vi "Normalize Waveform.vi"(0 "Waveform In":T1={"Waveform Name"="Wfm", "Waveform"={"x0"=0.0, "dx"=0.0, "y"=[]}, "Signal Bandwidth (Hz)"=0.0, "PAPR (dB)"=0.0, "Burst Length (s)"=0.0, "Sample Rate"=0.0, "Burst Start Locations"=[], "Burst Stop Locations"=[], "Idle Duration Present?"=FALSE} {"Sample Rate" format="%#_6p"; "Burst Length (s)" format="%#_6p"; "PAPR (dB)" format="%.2f"; "Signal Bandwidth (Hz)" format="%.2f"; "Waveform"."y" format="%.2f"; "Waveform"."dx" format="%^.2e"; "Waveform"."x0" format="%^.2e"}) -> (4 "Waveform Out":T1={"Waveform Name"="Wfm", "Waveform"={"x0"=0.0, "dx"=0.0, "y"=[]}, "Signal Bandwidth (Hz)"=0.0, "PAPR (dB)"=0.0, "Burst Length (s)"=0.0, "Sample Rate"=0.0, "Burst Start Locations"=[], "Burst Stop Locations"=[], "Idle Duration Present?"=FALSE} {"Sample Rate" format="%#_6p"; "Burst Length (s)" format="%#_6p"; "PAPR (dB)" format="%.2f"; "Signal Bandwidth (Hz)" format="%.2f"; "Waveform"."y" format="%.2f"; "Waveform"."dx" format="%^.2e"; "Waveform"."x0" format="%^.2e"})   [LabVIEW 2018, in "SG.lvlib"]
uses:
  SG.lvlib
  Typedefs/Waveform.ctl
  <vilib>/Analysis/5stat.llb/RMS (CDB).vi
  <vilib>/Analysis/NI_AALPro.lvlib
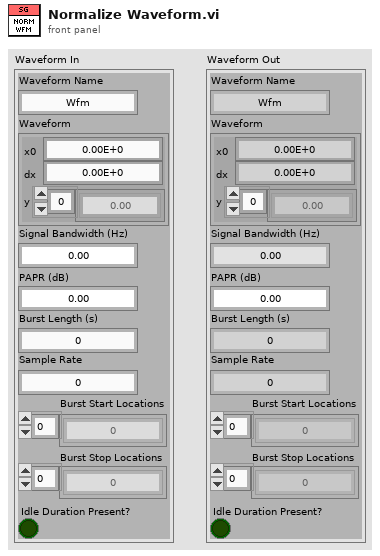
[diagram p1: front panel]
types:
  T1 = typedef "SG.lvlib/Waveform.ctl" = cluster{"Waveform Name":string, "Waveform":cluster{"x0":dbl, "dx":dbl, "y":csg[]}, "Signal Bandwidth (Hz)":dbl, "PAPR (dB)":dbl, "Burst Length (s)":dbl, "Sample Rate":dbl, "Burst Start Locations":i32[], "Burst Stop Locations":i32[], "Idle Duration Present?":bool}
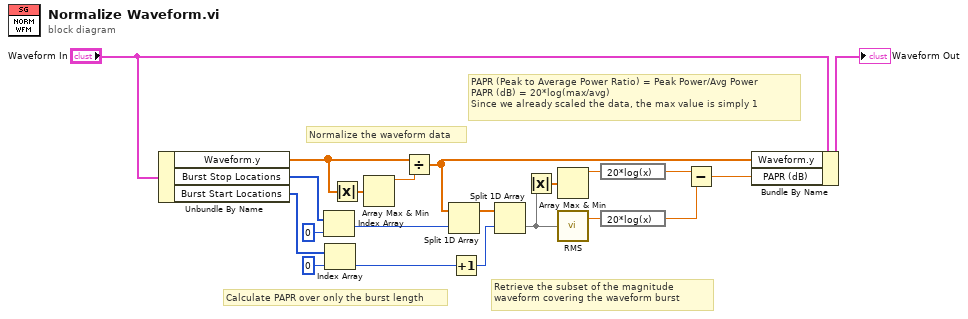
[diagram p0: block diagram]
diagram:
  # "PAPR (Peak to Average Power Ratio) = Peak Power/Avg Power\nPAPR (dB) = 20*log(max/avg)\nSince we already scaled the data, the max value is simply 1"
  # "Retrieve the subset of the magnitude waveform covering the waveform burst"
  # "Calculate PAPR over only the burst length"
  # "Normalize the waveform data"
  n1 = Unbundle By Name("Waveform In") -> ("Waveform.y"=w11:csg[], "Burst Stop Locations"=w20:i32[], "Burst Start Locations"=w19:i32[])
  n2 = Index Array(array=w20, index=0) -> (element=w3:i32)
  n3 = Index Array(array=w19, index=0) -> (element=w2:i32)
  n4 = Absolute Value(x=w11) -> (abs(x)=w16:sgl[])
  n5 = Array Max & Min(array=w16) -> (max value=w12:sgl)  [unwired: 3 out]
  n6 = Divide(x=w11, y=w12) -> (x/y=w4:csg[])
  n7 = Split 1D Array(array=w4, index=w3) -> (first subarray=w10:csg[])  [unwired: 1 out]
  n8 = Increment(x=w2) -> (x+1=w13:i32)
  n9 = Split 1D Array(array=w10, index=w13) -> (second subarray=w5:csg[])  [unwired: 1 out]
  n10 = Absolute Value(x=w5) -> (abs(x)=w9:sgl[])
  n11 = Array Max & Min(array=w9) -> (max value=w8:sgl)  [unwired: 3 out]
  n12 = call-poly <vilib>:"RMS.vi"("X"=w5) -> ("rms value"=w17:dbl)  [unwired: 1 out]
  n13 = expression code="20*log(x)"(w8) -> (w15:sgl)
  n14 = expression code="20*log(x)"(w17) -> (w1:dbl)
  n15 = Subtract(x=w15, y=w1) -> (x-y=w7:dbl)
  n16 = Bundle By Name(cluster="Waveform In", "Waveform.y"=w4, "PAPR (dB)"=w7) -> (→"Waveform Out":T1)
